vi "Third Ex.vi"() -> ()   [LabVIEW 2016]
panel:
  out "Loops":i32
  in  "stop":bool
  out "Boolean 2":bool
  out "Meter":dbl(knob) scale=-1.0..10.0
  in  "Boolean":bool
  in  "Knob":dbl(knob) scale=0.0..10.0
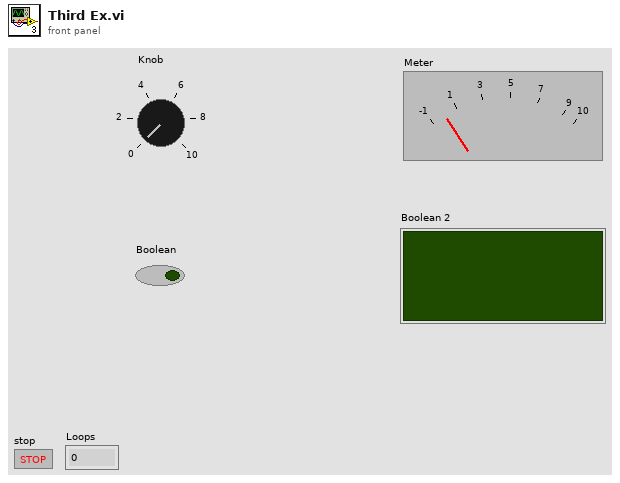
[diagram p1: front panel]
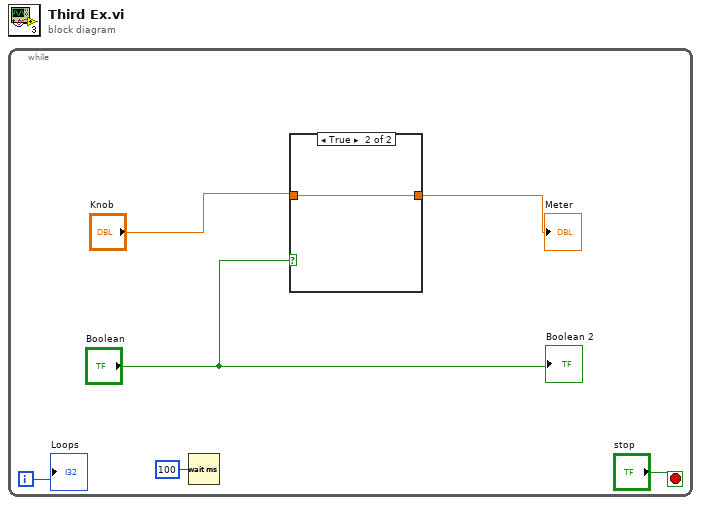
[diagram p0: block diagram]
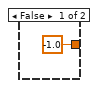
[diagram p2: hidden frame]
diagram:
  n1 = while {
    i -> [w2]
    stop <- "stop" stop-if-true
    n2 = Wait (ms)(milliseconds to wait=u32 100) -> ()  [unwired: 1 out]
    n3 = case shown="True" "Boolean" {
      tunnel: "Knob" -> [_ w8]
      tunnel: [-1.0 ("Knob") w8] -> w5
      frame False {
      }
      frame True {
      }
    }
    "Meter" <- w5
    "Boolean 2" <- "Boolean"
    "Loops" <- w2
  }
